vi "Charging_Extract Charging Status From String.vi"(11 "Charging Status":string="ChargingState=CHARGE_OFF-0\r\nChargeWarning=YES\r\nTemperatureLevel=35.4DEGREES\r\nIPG_ReceivedLevel=113") -> (0 "IPG_ReceivedLevel":dbl=nan, 1 "TemperatureLevel":dbl=nan, 2 "ChargeWarning":dbl=nan, 3 "ChargingState":string)   [LabVIEW 2020]
doc: "This function parses an IPG Telemetry Charging Status string into four parameters (one string and three double precision floating point data types).\n\nIf the status string format is incorrect, <not available> and NaN values will be returned."
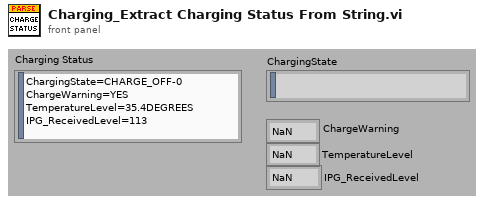
[diagram p1: front panel]
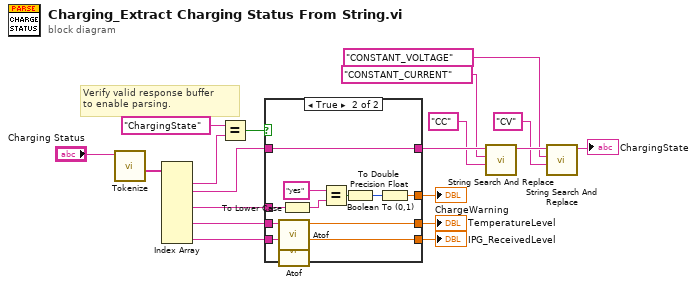
[diagram p0: block diagram]
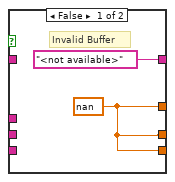
[diagram p2: hidden frame]
diagram:
  # "Verify valid response buffer\nto enable parsing."
  n1 = call "Tokenize.vi"("input string"="Charging Status") -> ("tokens"=w1:string[])  [unwired: 4 in, 2 out]
  n2 = Index Array(array=w1) -> (element #1=w13:string, element #2=w10:string, element #4=w17:string, element #6=w16:string, element #8=w15:string)  [unwired: 8 in, 3 out]
  n3 = Equal?(x="ChargingState", y=w13) -> (x = y?=w11:bool)
  n4 = case shown="True" w11 {
    tunnel: [w20 w30] -> w19
    tunnel: [w20 w29] -> w18
    tunnel: w17 -> [_ w28]
    tunnel: w16 -> [_ w27]
    tunnel: w15 -> [_ w26]
    tunnel: [w20 w23] -> w14
    tunnel: ["<not available>" ("token string") w22] -> w7
    tunnel: w10 -> [_ w22]
    frame False {
      w20 = nan
      # "Invalid Buffer"
    }
    frame True {
      n5 = call "Atof.vi"("string"=w27) -> ("number"=w30:dbl)  [unwired: 6 in]
      n6 = call "Atof.vi"("string"=w26) -> ("number"=w29:dbl)  [unwired: 6 in]
      n7 = To Lower Case(string=w28) -> (all lower case string=w25:string)
      n8 = Equal?(x="yes", y=w25) -> (x = y?=w31:bool)
      n9 = Boolean To (0,1)(Boolean=w31) -> (0, 1=w24:i16)
      n10 = To Double Precision Float(number=w24) -> (double precision float=w23:dbl)
    }
  }
  "ChargeWarning" <- w14
  "TemperatureLevel" <- w19
  "IPG_ReceivedLevel" <- w18
  n11 = call "String Search And Replace.vi"("replace with"="CC", "search for"="CONSTANT_CURRENT", "string in"=w7) -> ("string out"=w9:string)  [unwired: 5 in, 1 out]
  n12 = call "String Search And Replace.vi"("replace with"="CV", "search for"="CONSTANT_VOLTAGE", "string in"=w9) -> ("string out"=→"ChargingState":string)  [unwired: 5 in, 1 out]
